vi "6- 2D Array of random number.vi"() -> ()   [LabVIEW 2019]
panel:
  in  "?":bool
  in  "Number of column":i32
  in  "Number of row":i32
  out "?":string[](array[string])
  out "Array":dbl[][](array[numeric]) format="%#_3g"
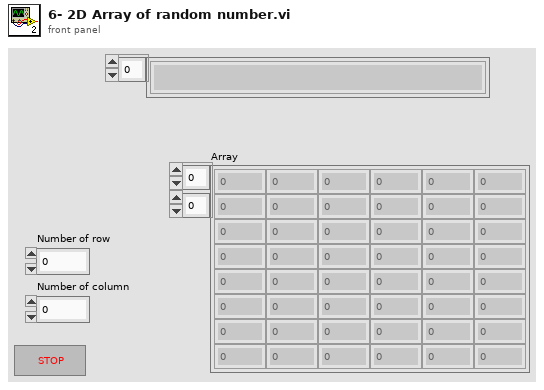
[diagram p1: front panel]
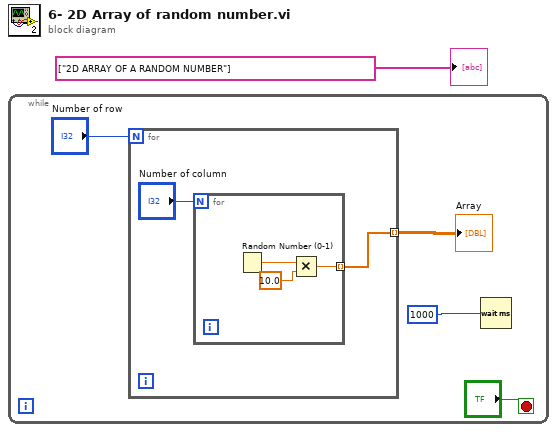
[diagram p0: block diagram]
diagram:
  n1 = while {
    stop <- "?" stop-if-true
    n2 = for {
      N: "Number of row" -> [_]
      tunnel: [w7] -> w5 mode=indexing
      n3 = for {
        N: "Number of column" -> [_]
        tunnel: [w9] -> w7 mode=indexing
        n4 = Random Number (0-1)() -> (number: 0 to 1=w10:dbl)
        n5 = Multiply(x=w10, y=10.0 ("x*y")) -> (x*y=w9:dbl)
      }
    }
    "Array" <- w5
    n6 = Wait (ms)(milliseconds to wait=u32 1000 ("millisecond timer value")) -> ()  [unwired: 1 out]
  }
  "?" <- string[] ["2D ARRAY OF A RANDOM NUMBER"] ("Array 2")
